vi "2100_Measure V and Publish.vi"(7 "Publishable ID":string="PreFuse_VIO", 8 "Error In":errorcluster, 10 "Pins":string[](array[string])=["VDD"], 11 "Semiconductor Module Context":T1) -> (0 "Error Out":errorcluster)   [LabVIEW 2013]
uses:
  <vilib>/NI_TestStand_SemiconductorModule/NI_TestStand_Semiconductor_Module.lvlibp/PinMap/General/SemiconductorModuleContext.ctl
  <vilib>/NI_TestStand_SemiconductorModule/NI_TestStand_Semiconductor_Module.lvlibp/PinMap/DC Power/PinsToNIDCPowerSessions.vi
  <vilib>/NI_TestStand_SemiconductorModule/NI_TestStand_Semiconductor_Module.lvlibp/PinMap/General/Publish/PublishDataDouble2D.vi
  <vilib>/NI_TestStand_SemiconductorModule/NI_TestStand_Semiconductor_Module.lvlibp
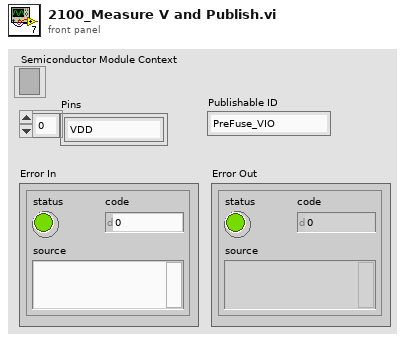
[diagram p1: front panel]
types:
  T1 = typedef "NI_TestStand_Semiconductor_Module.lvlibp/SemiconductorModuleContext.ctl" = refnum<k7>
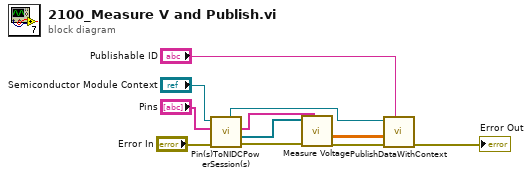
[diagram p0: block diagram]
diagram:
  n1 = call-poly <vilib>:"Pin(s)ToNIDCPowerSession(s).vi"("error in (no error)"="Error In", "Pins"="Pins", "Semiconductor Module Context"="Semiconductor Module Context") -> ("error out"=w11:errorcluster, "Instrument Sessions"=w10:refnum<k15>[], "Channel Lists"=w9:string[], "Pin Query Context"=w5:refnum<class "MultiplePinMultipleSessionQueryContext.lvclass">)  [unwired: 4 in, 1 out]
  n2 = call "Measure Voltage.vi"("Channel Lists"=w9, "error in (no error)"=w11, "DCPower Sessions In"=w10) -> ("error out"=w3:errorcluster, "Voltage measurements"=w4:dbl[][])  [unwired: 6 in, 1 out]
  n3 = call-poly <vilib>:"PublishDataWithContext.vi"("Published Data Id"="Publishable ID", "error in (no error)"=w3, "Data In"=w4, "Pin Query Context"=w5) -> ("error out"=→"Error Out":errorcluster)  [unwired: 6 in, 1 out]
